vi "Query Event Log All Entries.vi"(8 "error in (no error)":errorcluster, 11 "VISA resource name":refnum<visa-resource-name>) -> (0 "error out":errorcluster, 2 "Event Logs":T1(array[cluster]), 3 "VISA resource name out":refnum<visa-resource-name>)   [LabVIEW 2015, in "Rohde&Schwarz CMXP Base.lvlib"]
doc: "Queries all event log entries.\n\nAttribute:\nRSCMXPBASE_ATTR_EVENT_LOG_ALL_ENTRIES\n\nRemote-control command:\nSENSe:ELOG:ALL?"
uses:
  <instrlib>/Rohde&Schwarz CMXP Base/Rohde&Schwarz CMXP Base.lvlib
  <instrlib>/Rohde&Schwarz CMXP Base/Private/rsidr_core.llb/rsidr_core.lvlib
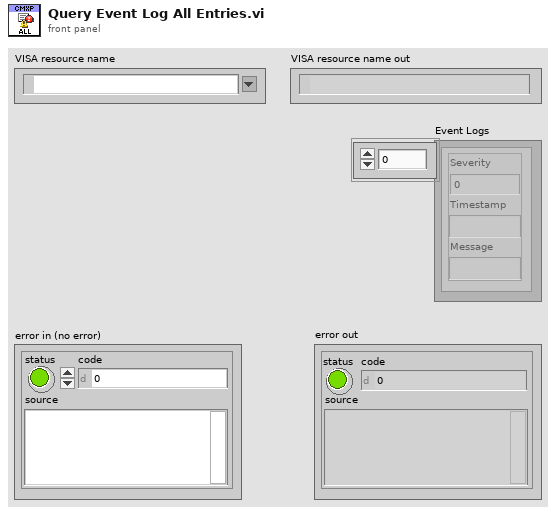
[diagram p1: front panel]
types:
  T1 = cluster{"Severity":dbl, "Timestamp":string, "Message":string}[]
  T2 = cluster{"Severity":i32, "Timestamp":string, "Message":string}
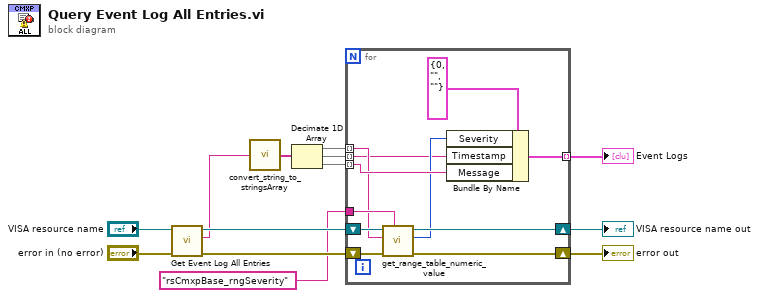
[diagram p0: block diagram]
diagram:
  n1 = call "Get Event Log All Entries"("error in (no error)"="error in (no error)", "instrument handle"="VISA resource name") -> ("error out"=w6:errorcluster, "Event Log All Entries"=w1:string, "instrument handle out"=w5:refnum<visa-resource-name>)  [unwired: 7 in]
  n2 = call <instrlib>:"convert_string_to_stringsArray.vi"("String in"=w1) -> ("string array out"=w11:string[])  [unwired: 3 in, 1 out]
  n3 = Decimate 1D Array(w11) -> (w10:string[], w9:string[], w8:string[])
  n4 = for {
    tunnel: w10 -> [w16] mode=indexing
    tunnel: w9 -> [w14] mode=indexing
    tunnel: w8 -> [w23] mode=indexing
    tunnel: [w22] -> w7 mode=indexing
    tunnel: "rsCmxpBase_rngSeverity" ("Range Table ID in") -> [w19]
    shift-right: [w17] -> w4
    shift-left: w5 -> [w20]
    shift-right: [w18] -> w3
    shift-left: w6 -> [w21]
    n5 = call <instrlib>:"get_range_table_numeric_value.vi"("Range Table ID in"=w19, "error in"=w21, "String Value"=w16, "VISA resource name"=w20) -> ("error out"=w18:errorcluster, "I32 output"=w15:i32, "VISA resource name out"=w17:refnum<visa-resource-name>)  [unwired: 5 in]
    n6 = Bundle By Name(cluster=T2 {"Severity"=0, "Timestamp"="", "Message"=""} ("Event Logs 2"), "Severity"=w15, "Timestamp"=w14, "Message"=w23) -> (w22:T2)
  }
  "error out" <- w3
  "VISA resource name out" <- w4
  "Event Logs" <- w7
